vi "TDMS Advanced Set Waveform Properties.vi"(8 "error in (no error)":errorcluster, 9 "Waveform":waveform(dbl)={"t0"=timestamp(0 s since 1904-01-01), "dt"=0.0, "Y"=[]}, 10 "group name":string, 11 "tdms file":refnum<k34>) -> (0 "error out":errorcluster, 1 "channel name out":string, 2 "group name out":string, 3 "tdms file out":refnum<k34>, 4 "samples per channel":i32)   [LabVIEW 2019]
doc: "Set TDMS Waveform Properties."
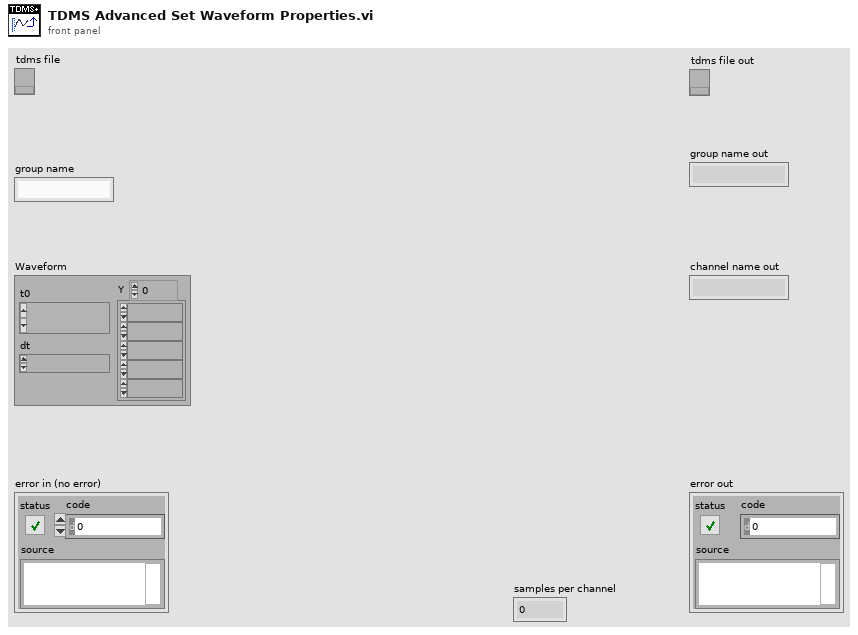
[diagram p1: front panel]
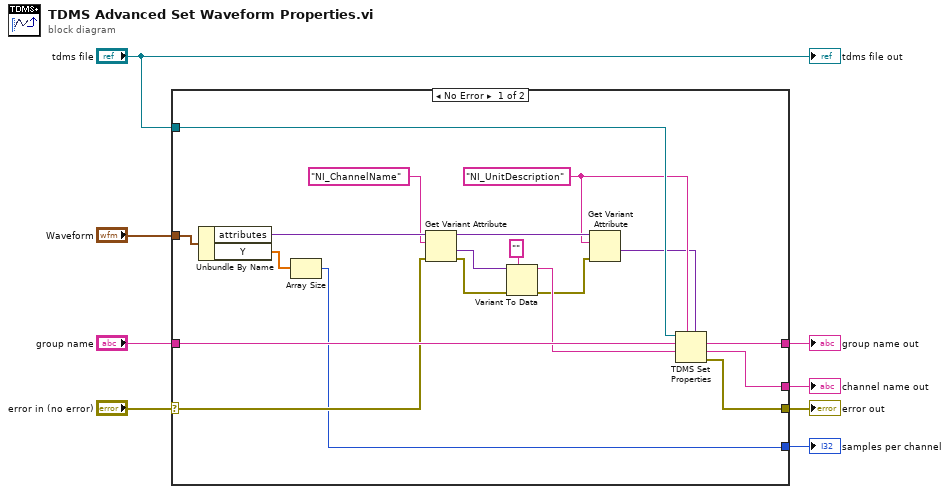
[diagram p0: block diagram]
diagram:
  n1 = case shown="No Error" "error in (no error)" {
    selector: "error in (no error)" -> [w11 w29]
    tunnel: "group name" -> [w27 w28]
    tunnel: "tdms file" -> [w26 _]
    tunnel: [w25 w29] -> w7
    tunnel: [w24 _] -> w6
    tunnel: [w23 w28] -> w5
    tunnel: "Waveform" -> [w17 _]
    tunnel: [w9 _] -> w1
    frame No Error {
      w13 = "NI_UnitDescription" ("name")
      n2 = Unbundle By Name(w17) -> ("attributes"=w22:variant, "Y"=w10:dbl[])
      n3 = Array Size(array=w10) -> (size(s)=w9:i32)
      n4 = Get Variant Attribute(Variant=w22, name="NI_ChannelName", error in=w11) -> (duplicate Variant=w14:variant, value=w19:variant, error out=w18:errorcluster)  [unwired: 1 in, 1 out]
      n5 = Variant To Data(error in=w18, type="", Variant=w19) -> (data=w16:string, error out=w15:errorcluster)
      n6 = Get Variant Attribute(Variant=w14, name=w13, error in=w15) -> (value=w12:variant)  [unwired: 1 in, 3 out]
      n7 = TDMS Set Properties(5:w12, 7:w13, 9:w16, 10:w27, 11:w26) -> (0:w25:errorcluster, 1:w24:string, 2:w23:string)  [unwired: 1 in, 1 out]
    }
    frame Error {
    }
  }
  "error out" <- w7
  "channel name out" <- w6
  "group name out" <- w5
  "samples per channel" <- w1
  "tdms file out" <- "tdms file"
